vi "Two devices.vi"() -> ()   [LabVIEW 2015]
doc: "This example VI shows how to convert string data elements to numeric elements so it can be graphed and displayed on an XY Graph."
uses:
  <instrlib>/Keithley 27XX/Public/Configure/Measurement Specific/Configure Thermocouple.vi
  <instrlib>/Keithley 27XX/Keithley 27XX.lvlib
panel:
  out "Cryocon Temp":dbl(graph)
  in  "Set Input":u8(ring) items=["ChA", "ChB", "ChC", "ChD"]
  in  "error in (no error)":errorcluster
  in  "baud rate (9600)":u32=9600
  in  "Port":string="10::INSTR"
  in  "Interface":u16(ring) items=["GPIB", "Serial"]
  in  "Save File?":bool
  out "Waveform Chart 3":dbl[](graph)
  out "Waveform Chart 2":dbl[](graph)
  out "Waveform Chart":dbl[](graph)
  in  "Enable Open Detector? (False)":bool
  in  "Simulated Reference Temperature (23 deg C)":dbl=23.0
  in  "Reference Junction Type (0: Simulated)":u16(ring)=1 items=["Simulated", "Internal", "External"]
  in  "Thermocouple Type (1: K)":u16(ring)=1 items=["J", "K", "T", "E", "R", "S", "B", "N"]
  in  "Column headers":string[](array[string])=["Time/s", "TH/Celsius", "TC/Celsius", "Delta V"]
  in  "Number of channels":i32=1
  in  "Pause/Continue":bool
  in  "stop":bool
  out "Numeric":i32
  out "concatenated string":string
  in  "file (use dialog)":path=path "C:/Users/Guest_2/Desktop/Zong Long/Data trial.txt"
  in  "Function (6: Temp)":u16(ring)=6 items=["DC Voltage", "AC Voltage", "DC Current", "AC Current", "Resistance", "Four-Wire Resistance", "Temperature (C)", "Frequency", "Period", "Continuity"]
  in  "Channel List (101)":string="101"
  in  "Serial Configuration":T1={"Baud Rate (9600)"=9600, "Flow Control (1: XON/XOFF)"=1, "Termination Char (0:CR)"=0} {"Termination Char (0:CR)" items=["CR", "LF", "CRLF (Do not use)", "LFCR (Do not use)"]; "Flow Control (1: XON/XOFF)" items=["None", "XON/XOFF", "RTS/CTS (2701 Only)", "XON/XOFF & RTS/CTS (2701 Only)"]; "Baud Rate (9600)" items=["300"=300, "600"=600, "1200"=1200, "2400"=2400, "4800"=4800, "9600"=9600, "19.2k"=19200, "38.4k (2701 Only)"=38400, "57.6k (2701 Only)"=57600, "115.2k (2701 Only)"=115200]}
  in  "Keithley VISA \nresource name":refnum<visa-resource-name>="GPIB0::19::INSTR"
  # "Keithley INIT"
  # "Cryocon INIT"
  # "Remember to change the number of channels"
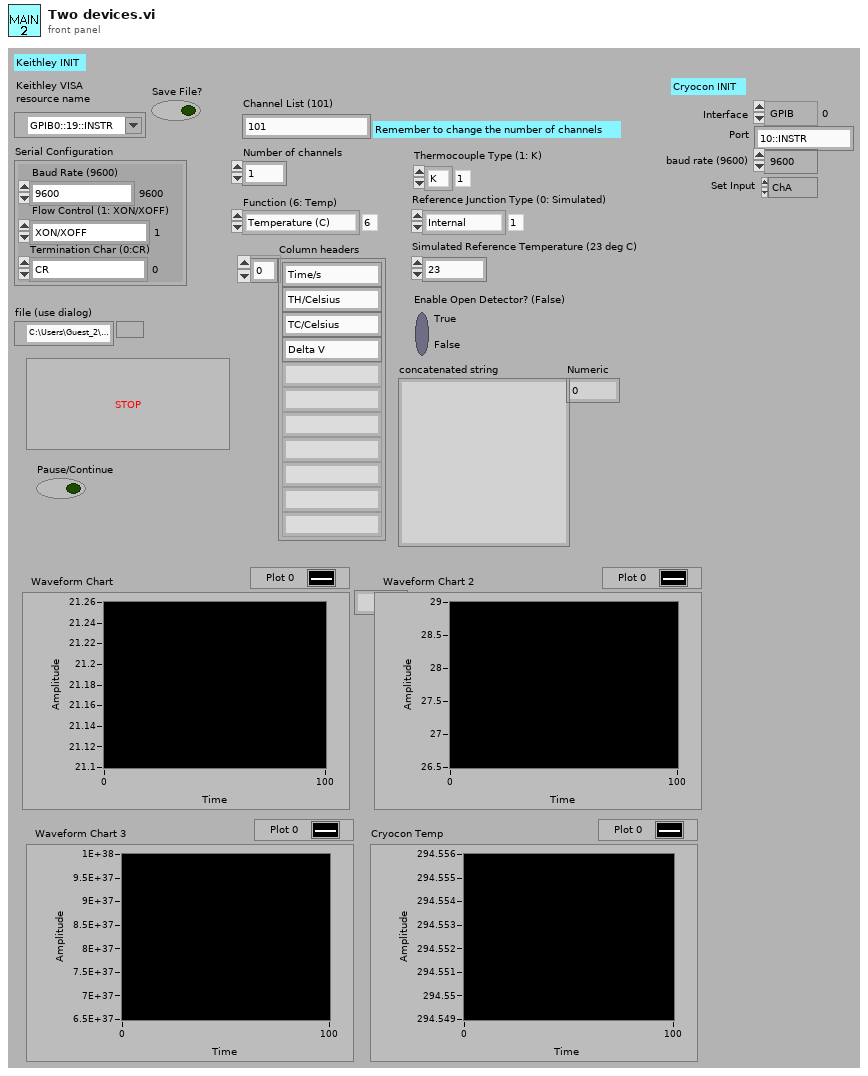
[diagram p1: front panel]
types:
  T1 = cluster{"Baud Rate (9600)":u32, "Flow Control (1: XON/XOFF)":u16, "Termination Char (0:CR)":u16}
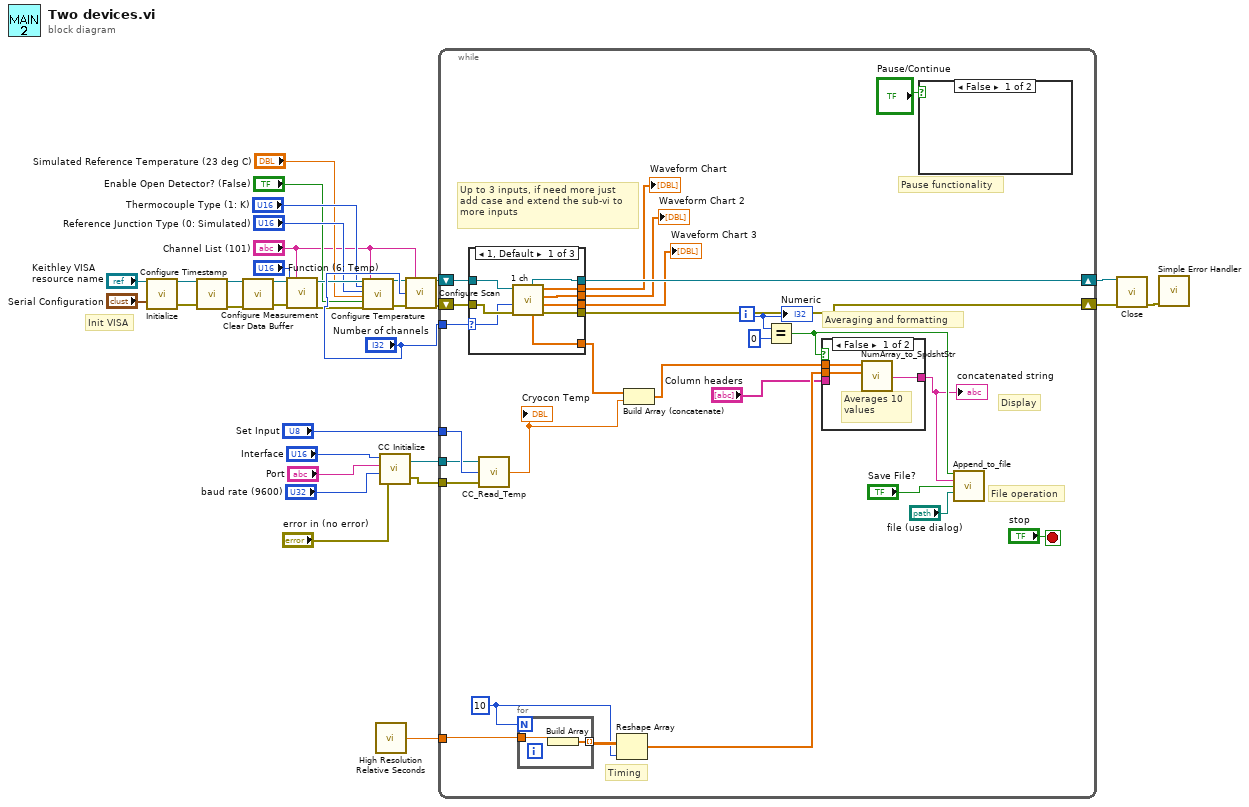
[diagram p0: block diagram]
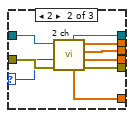
[diagram p2: hidden frame]
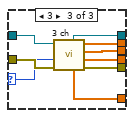
[diagram p3: hidden frame]
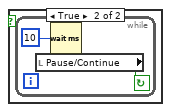
[diagram p4: hidden frame]
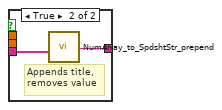
[diagram p5: hidden frame]
diagram:
  # "Init VISA"
  n1 = call <instrlib>:"Initialize.vi"("VISA resource name"="Keithley VISA \nresource name", "Serial Configuration"="Serial Configuration") -> ("VISA resource name out"=w29:refnum<visa-resource-name>, "error out"=w28:errorcluster)  [unwired: 12 in]
  n2 = call <instrlib>:"Configure Timestamp.vi"("VISA resource name"=w29, "error in (no error)"=w28) -> ("VISA resource name out"=w24:refnum<visa-resource-name>, "error out"=w23:errorcluster)  [unwired: 12 in]
  n3 = call <instrlib>:"Clear Data Buffer.vi"("VISA resource name"=w24, "error in (no error)"=w23) -> ("VISA resource name out"=w22:refnum<visa-resource-name>, "error out"=w25:errorcluster)  [unwired: 12 in]
  n4 = call <instrlib>:"Configure Measurement.vi"("VISA resource name"=w22, "Scan List (Empty)"="Channel List (101)", "Function (0: DC Voltage)"="Function (6: Temp)", "error in (no error)"=w25) -> ("VISA resource name out"=w16:refnum<visa-resource-name>, "error out"=w13:errorcluster)  [unwired: 10 in]
  n5 = call-poly <instrlib>:"Configure Temperature.vi"("VISA resource name"=w16, "Thermocouple Type (1: K)"="Thermocouple Type (1: K)", "Reference Junction Type (0: Simulated)"="Reference Junction Type (0: Simulated)", "Simulated Reference Temperature (23 deg C)"="Simulated Reference Temperature (23 deg C)", "Enable Open Detector? (False)"="Enable Open Detector? (False)", "error in (no error)"=w13, "Scan List (Empty)"="Channel List (101)") -> ("VISA resource name out"=w15:refnum<visa-resource-name>, "error out"=w14:errorcluster)  [unwired: 11 in]
  n6 = call <vilib>:"High Resolution Relative Seconds.vi"() -> ("relative seconds"=w18:dbl)
  n7 = call "CC Initialize.vi"("error in (no error)"="error in (no error)", "baud rate (9600)"="baud rate (9600)", "Port"="Port", "Interface"="Interface") -> ("error out"=w1:errorcluster, "VISA out"=w2:refnum<visa-resource-name>)
  n8 = call <instrlib>:"Configure Scan.vi"("VISA resource name"=w15, "Channel List (101:110)"="Channel List (101)", "Sample Count (100)"="Number of channels", "error in (no error)"=w14) -> ("VISA resource name out"=w20:refnum<visa-resource-name>, "error out"=w19:errorcluster)  [unwired: 10 in]
  n9 = while {
    shift-right: [w58] -> w26
    shift-left: w20 -> [w57]
    shift-right: [w59] -> w27
    shift-left: w19 -> [w56]
    tunnel: w18 -> [w54]
    tunnel: "Number of channels" -> [w47]
    tunnel: "Set Input" -> [w38]
    tunnel: w2 -> [w37]
    tunnel: w1 -> [w36]
    i -> [w49]
    stop <- "stop" stop-if-true
    w46 = 10 ("x")
    # "Timing"
    # "Up to 3 inputs, if need more just\nadd case and extend the sub-vi to\nmore inputs"
    # "Display"
    # "Averaging and formatting"
    # "File operation"
    # "Pause functionality"
    n10 = case shown="1, Default" w47 {
      selector: w47 -> [w67 w74 w83]
      tunnel: [w63 w75 w84] -> w59
      tunnel: [w65 w72 w82] -> w58
      tunnel: w57 -> [w66 w77 w85]
      tunnel: w56 -> [w68 w76 w86]
      tunnel: [w62 w70 w80] -> w43
      tunnel: [w61 w71 w79] -> w45
      tunnel: [w60 w73 w78] -> w44
      tunnel: [w64 w69 w81] -> w35
      frame 1, Default {
        n11 = call "1 ch.vi"("error out"=w68, "Number of channels"=w67, "VISA resource name out"=w66) -> ("error out 2"=w63:errorcluster, "output array 3"=w60:dbl[], "output array 2"=w61:dbl[], "Means of 10"=w62:dbl[], "output array"=w64:dbl[], "VISA resource name out 2"=w65:refnum<visa-resource-name>)  [unwired: 3 in]
      }
      frame 2 {
        n12 = call "2 ch.vi"("error out"=w76, "Number of channels"=w74, "VISA resource name out"=w77) -> ("error out 2"=w75:errorcluster, "Means of 12"=w73:dbl[], "Means of 11"=w71:dbl[], "Means of 10"=w70:dbl[], "output array"=w69:dbl[], "VISA resource name out 2"=w72:refnum<visa-resource-name>)  [unwired: 3 in]
      }
      frame 3 {
        n13 = call "3 ch.vi"("error out"=w86, "Number of channels"=w83, "VISA resource name out"=w85) -> ("error out 2"=w84:errorcluster, "Means of 12"=w78:dbl[], "Means of 11"=w79:dbl[], "Means of 10"=w80:dbl[], "output array"=w81:dbl[], "VISA resource name out 2"=w82:refnum<visa-resource-name>)  [unwired: 3 in]
      }
    }
    "Waveform Chart 3" <- w44
    "Waveform Chart 2" <- w45
    "Waveform Chart" <- w43
    n14 = call "CC_Read_Temp.vi"("error in (no error)"=w36, "Input"=w38, "VISA In"=w37) -> ("Temperature"=w34:dbl)  [unwired: 2 out]
    "Cryocon Temp" <- w34
    n15 = for {
      N: w46 -> [_]
      tunnel: w54 -> [w90]
      tunnel: [w89] -> w53 mode=indexing
      n16 = Build Array(w90) -> (w89:dbl[])
    }
    n17 = Reshape Array(w53, w46) -> (w52:dbl[])
    n18 = Build Array (concatenate)(w35, w34) -> (w33:dbl[])
    n19 = Equal?(x=w49, y=0) -> (x = y?=w41:bool)
    n20 = case shown="False" w41 {
      tunnel: w33 -> [w93 _]
      tunnel: w52 -> [w92 _]
      tunnel: [w91 w95] -> w40
      tunnel: "Column headers" -> [_ w94]
      frame False {
        # "Averages 10 \nvalues"
        n21 = call "NumArray_to_SpdshtStr.vi"("element 2"=w92, "element"=w93) -> ("concatenated string"=w91:string)  [unwired: 8 in, 1 out]
      }
      frame True {
        # "Appends title,\nremoves value"
        n22 = call "NumArray_to_SpdshtStr_prepend.vi"("Column headers"=w94) -> ("concatenated string"=w95:string)  [unwired: 10 in]
      }
    }
    "concatenated string" <- w40
    n23 = case shown="False" "Pause/Continue" {
      frame False {
      }
      frame True {
        n24 = while {
          stop <- w88 continue-if-true
          n25 = local read "Pause/Continue"() -> (w88:bool)
          n26 = Wait (ms)(milliseconds to wait=u32 10) -> ()  [unwired: 1 out]
        }
      }
    }
    n27 = call "Append_to_file.vi"("Boolean"=w41, "text"=w40, "Save File?"="Save File?", "file path (use dialog)"="file (use dialog)") -> ()  [unwired: 11 in, 1 out]
    "Numeric" <- w49
  }
  n28 = call <instrlib>:"Close.vi"("VISA resource name"=w26, "error in (no error)"=w27) -> ("error out"=w30:errorcluster)  [unwired: 13 in]
  n29 = call <vilib>:"Simple Error Handler.vi"("error in (no error)"=w30) -> ()  [unwired: 4 in, 5 out]
